vi "test_EnumerateServices_StopDiscoveryService_EnumerateServicesWorkWithoutError.vi"(8 "error in":errorcluster) -> (0 "error out":errorcluster, 2 "result":string, 3 "pass":bool)   [LabVIEW 2021, in "MeasurementServerTests.lvlib" / "Discovery Tests.lvlib"]
uses:
  Discovery Tests.lvlib
  gRPC/Generated APIs/ni/measurementlink/discovery/v1/RPC Messages/ni_measurementlink_discovery_v1_EnumerateServicesRequest.ctl
  MeasurementServerTests.lvlib
  gRPC/Generated APIs/ni/measurementlink/discovery/v1/ni.measurementlink.discovery.v1.api.lvlib
  Runtime/Clients/Discovery V1/NI Discovery V1 Client.lvlib
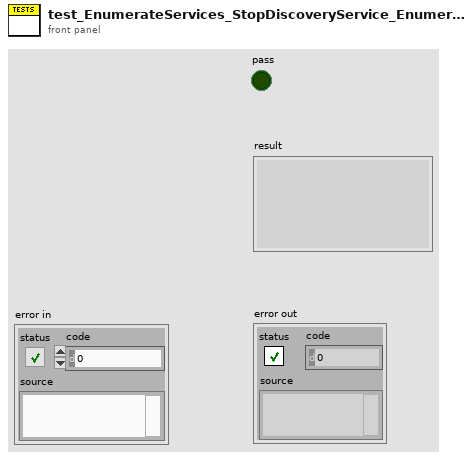
[diagram p1: front panel]
types:
  T1 = typedef "ni.measurementlink.discovery.v1.api.lvlib/ni_measurementlink_discovery_v1_EnumerateServicesRequest.ctl" = cluster{"provided_interface":string}
  T2 = typedef "ni.measurementlink.discovery.v1.api.lvlib/ni_measurementlink_discovery_v1_EnumerateServicesResponse.ctl" = cluster{"available_services":T3[]}
  T3 = typedef "ni.measurementlink.discovery.v1.api.lvlib/ni_measurementlink_discovery_v1_ServiceDescriptor.ctl" = cluster{"display_name":string, "description_url":string, "provided_interfaces":string[], "service_class":string, "annotations":T4[]}
  T4 = typedef "ni.measurementlink.discovery.v1.api.lvlib/ni_measurementlink_discovery_v1_ServiceDescriptor_AnnotationsEntry.ctl" = cluster{"key":string, "value":string}
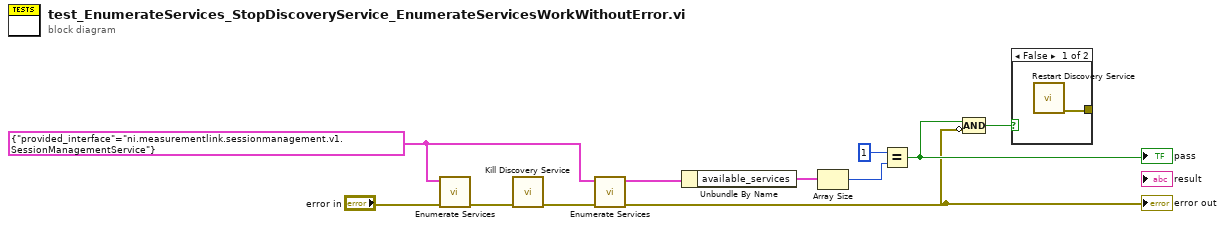
[diagram p0: block diagram]
diagram:
  w1 = T1 {"provided_interface"="ni.measurementlink.sessionmanagement.v1.SessionManagementService"} ("request data")
  n1 = call "Enumerate Services.vi"("error in"="error in", "request data"=w1) -> ("error out"=w5:errorcluster)  [unwired: 7 in, 1 out]
  n2 = call "Kill Discovery Service.vi"("error in"=w5) -> ("error out"=w4:errorcluster)  [unwired: 10 in]
  n3 = call "Enumerate Services.vi"("error in"=w4, "request data"=w1) -> ("error out"=w3:errorcluster, "response data"=w2:T2)  [unwired: 7 in]
  "error out" <- w3
  n4 = Unbundle By Name(w2) -> ("available_services"=w9:T3[])
  n5 = Array Size(array=w9) -> (size(s)=w8:i32)
  n6 = Equal?(x=1, y=w8) -> (x = y?=w6:bool)
  "pass" <- w6
  n7 = Compound Arithmetic op=AND(w6, invert w3) -> (w10:bool)
  n8 = case shown="False" w10 {
    tunnel: [w12 _] -> _
    frame False {
      n9 = call "Restart Discovery Service.vi"() -> ("error out"=w12:errorcluster)  [unwired: 11 in]
    }
    frame True {
    }
  }
